vi "rsidr_core_global.vi"() -> ()   [LabVIEW 2020, in "Rohde&Schwarz RTx Oscilloscopes.lvlib"] (continued)
"Access"=2, "Range Table"="", "Read Callback"="", "Write Callback"="", "Supported Models"="", "Instrument Options"="", "Flags"=0, "Help"="If persistence is enabled (DISPlay:PERSistence[:STATe]), each new data point in the diagram area remains on the screen infinitely until this command is set to OFF.\n\nAvailable Repeated Capabilities:\nNone\n\nRemote-control command(s):\nDISPlay:PERSistence:INFinite"}, {"Level"=3, "Class Only"=FALSE, "Identifier"="RSRTX_ATTR_PERSISTENCE_TIME", "Descriptive Name"="Persistence Time", "Data Type"=1, "Command"="DISP:PERS:TIME", "Access"=2, "Range Table"="", "Read Callback"="", "Write Callback"="", "Supported Models"="", "Instrument Options"="", "Flags"=0, "Help"="If persistence is enabled (DISPlay:PERSistence[:STATe]), each new data point in the diagram area remains on the screen for the duration defined here.\n\nAvailable Repeated Capabilities:\nNone\n\nRemote-control command(s):\nDISPlay:PERSistence:TIME"}, {"Level"=3, "Class Only"=FALSE, "Identifier"="RSRTX_ATTR_PERSISTENCE_CLEAR", "Descriptive Name"="Persistence Clear", "Data Type"=4, "Command"="DISP:PERS:CLE", "Access"=1, "Range Table"="", "Read Callback"="", "Write Callback"="", "Supported Models"="", "Instrument Options"="", "Flags"=0, "Help"="Removes the displayed persistent waveform from the screen.\n\nAvailable Repeated Capabilities:\nNone\n\nRemote-control command(s):\nDISPlay:PERSistence:CLEar"}, {"Level"=2, "Class Only"=TRUE, "Identifier"="", "Descriptive Name"="XY Diagram", "Data Type"=0, "Command"="", "Access"=0, "Range Table"="", "Read Callback"="", "Write Callback"="", "Supported Models"="", "Instrument Options"="", "Flags"=0, "Help"="Contains attributes for XY Diagram settings."}, {"Level"=3, "Class Only"=FALSE, "Identifier"="RSRTX_ATTR_XY_X_SOURCE", "Descriptive Name"="XY X Source", "Data Type"=0, "Command"="DISP:XY:XSO", "Access"=2, "Range Table"="rsrtx_rngSource", "Read Callback"="", "Write Callback"="", "Supported Models"="", "Instrument Options"="", "Flags"=0, "Help"="Defines the source to be displayed in x direction in an XY-diagram, replacing the usual time base.\n\nAvailable Repeated Capabilities:\nNone\n\nRemote-control command(s):\nDISPlay:XY:XSOurce"}, {"Level"=3, "Class Only"=FALSE, "Identifier"="RSRTX_ATTR_XY_Y_SOURCE", "Descriptive Name"="XY Y Source", "Data Type"=0, "Command"="DISP:XY:Y1S", "Access"=2, "Range Table"="rsrtx_rngSource", "Read Callback"="", "Write Callback"="", "Supported Models"="", "Instrument Options"="", "Flags"=0, "Help"="Defines the (first) source to be displayed in y direction in an XY-diagram.\n\nAvailable Repeated Capabilities:\nNone\n\nRemote-control command(s):\nDISPlay:XY:Y1Source"}, {"Level"=3, "Class Only"=FALSE, "Identifier"="RSRTX_ATTR_XY_Y2_SOURCE", "Descriptive Name"="XY Y2 Source", "Data Type"=0, "Command"="DISP:XY:Y2S", "Access"=2, "Range Table"="rsrtx_rngXY2Source", "Read Callback"="", "Write Callback"="", "Supported Models"="", "Instrument Options"="", "Flags"=0, "Help"="Defines an optional second source to be displayed in y direction in an XY-diagram. Only relevant for 4-channel  instruments.\n\nAvailable Repeated Capabilities:\nNone\n\nRemote-control command(s):\nDISPlay:XY:Y2Source"}, {"Level"=3, "Class Only"=FALSE, "Identifier"="RSRTX_ATTR_XY_Z_SOURCE", "Descriptive Name"="XY Z Source", "Data Type"=0, "Command"="DISP:XY:ZSO", "Access"=2, "Range Table"="rsrtx_rngSource", "Read Callback"="", "Write Callback"="", "Supported Models"="", "Instrument Options"="", "Flags"=0, "Help"="Defines the source to be used to determine the intensity of the xy-waveform.\n\nAvailable Repeated Capabilities:\nNone\n\nRemote-control command(s):\nDISPlay:XY:ZSOurce"}, {"Level"=3, "Class Only"=FALSE, "Identifier"="RSRTX_ATTR_XY_Z_TRESHOLD", "Descriptive Name"="XY Z Treshold", "Data Type"=1, "Command"="DISP:XY:ZTHR", "Access"=2, "Range Table"="rsrtx_rngIntensityTreshold", "Read Callback"="", "Write Callback"="", "Supported Models"="", "Instrument Options"="", "Flags"=0, "Help"="Defines the threshold for intensity with a two-state modulation, if DISPlay: XY: ZMODe is set to DIGital.\n\nAvailable Repeated Capabilities:\nNone\n\nRemote-control command(s):\nDISPlay:XY:ZTHReshold"}, {"Level"=3, "Class Only"=FALSE, "Identifier"="RSRTX_ATTR_XY_INTENSITY_CONTROL", "Descriptive Name"="XY Intensity Control", "Data Type"=0, "Command"="DISP:XY:ZMOD", "Access"=2, "Range Table"="rsrtx_rngIntensityMode", "Read Callback"="", "Write Callback"="", "Supported Models"="", "Instrument Options"="", "Flags"=0, "Help"="Activates or deactivates the intensity control of the waveform via an additional signal source and sets the intensity mode.\n\nAvailable Repeated Capabilities:\nNone\n\nRemote-control command(s):\nDISPlay:XY:ZMODe"}, {"Level"=2, "Class Only"=TRUE, "Identifier"="", "Descriptive Name"="Zoom", "Data Type"=0, "Command"="", "Access"=0, "Range Table"="", "Read Callback"="", "Write Callback"="", "Supported Models"="", "Instrument Options"="", "Flags"=0, "Help"="Zoom definition."}, {"Level"=3, "Class Only"=FALSE, "Identifier"="RSRTX_ATTR_ZOOM_WINDOW_ENABLED", "Descriptive Name"="Zoom Window Enabled", "Data Type"=3, "Command"="TIM:ZOOM:STAT", "Access"=2, "Range Table"="", "Read Callback"="", "Write Callback"="", "Supported Models"="", "Instrument Options"="", "Flags"=0, "Help"="Switches the zoom window on or off.\n\nAvailable Repeated Capabilities:\nNone\n\nRemote-control command(s):\nTIMebase:ZOOM:STATe"}, {"Level"=3, "Class Only"=FALSE, "Identifier"="RSRTX_ATTR_ZOOM_DIAGRAM_TIMEBASE", "Descriptive Name"="Zoom Diagram Timebase", "Data Type"=1, "Command"="TIM:ZOOM:SCAL", "Access"=2, "Range Table"="", "Read Callback"="", "Write Callback"="", "Supported Models"="", "Instrument Options"="", "Flags"=0, "Help"="Defines the time base in the zoom diagram in seconds per division.\n\nAvailable Repeated Capabilities:\nNone\n\nRemote-control command(s):\nTIMebase:ZOOM:SCALe"}, {"Level"=3, "Class Only"=FALSE, "Identifier"="RSRTX_ATTR_ZOOM_OFFSET_OF_TRIGGER_POINT", "Descriptive Name"="Zoom Offset Of Trigger Point", "Data Type"=1, "Command"="TIM:ZOOM:TIME", "Access"=2, "Range Table"="", "Read Callback"="", "Write Callback"="", "Supported Models"="", "Instrument Options"="", "Flags"=0, "Help"="Defines the offset of the trigger point to the reference point of the zoom diagram.\n\nAvailable Repeated Capabilities:\nNone\n\nRemote-control command(s):\nTIMebase:ZOOM:TIME"}, {"Level"=3, "Class Only"=FALSE, "Identifier"="RSRTX_ATTR_ZOOM_REFERENCE_POINT", "Descriptive Name"="Zoom Reference Point", "Data Type"=1, "Command"="TIM:ZOOM:POS", "Access"=2, "Range Table"="rsrtx_rngPct", "Read Callback"="", "Write Callback"="", "Supported Models"="", "Instrument Options"="", "Flags"=0, "Help"="Defines the position of the zoom reference point (the reference point of the zoom window) in relation to the reference point of original time base.\n\nAvailable Repeated Capabilities:\nNone\n\nRemote-control command(s):\nTIMebase:ZOOM:POSition"}, {"Level"=3, "Class Only"=FALSE, "Identifier"="RSRTX_ATTR_ZOOM_WINDOW_POSITION", "Descriptive Name"="Zoom Window Position", "Data Type"=0, "Command"="DISP:CBAR:ZOOM", "Access"=2, "Range Table"="", "Read Callback"="", "Write Callback"="", "Supported Models"="", "Instrument Options"="", "Flags"=0, "Help"="Defines the position of the divide bar between normal waveform and zoom window. Sets the vertical position in pixels, measured from the top edge. The vertical display size is 800 px.\n\nAvailable Repeated Capabilities:\nNone\n\nRemote-control command(s):\nDISPlay:CBAR:ZOOM[:POSition]"}, {"Level"=3, "Class Only"=FALSE, "Identifier"="RSRTX_ATTR_ZOOM_SAMPLE_RATE", "Descriptive Name"="Zoom Sample Rate", "Data Type"=1, "Command"="ACQ:SRAT:ZOOM?", "Access"=0, "Range Table"="", "Read Callback"="", "Write Callback"="", "Supported Models"="", "Instrument Options"="", "Flags"=0, "Help"="Returns the sample rate of the zoom window.\n\nAvailable Repeated Capabilities:\nNone\n\nRemote-control command(s):\nACQuire:SRATe:ZOOM?"}, {"Level"=2, "Class Only"=TRUE, "Identifier"="", "Descriptive Name"="Markers", "Data Type"=0, "Command"="", "Access"=0, "Range Table"="", "Read Callback"="", "Write Callback"="", "Supported Models"="", "Instrument Options"="", "Flags"=0, "Help"="Markers configuration."}, {"Level"=3, "Class Only"=FALSE, "Identifier"="RSRTX_ATTR_MARKER_SET", "Descriptive Name"="Marker Set", "Data Type"=4, "Command"="TST:SET", "Access"=1, "Range Table"="", "Read Callback"="", "Write Callback"="", "Supported Models"="", "Instrument Options"="", "Flags"=0, "Help"="Sets a new marker (timestamp) at the reference point of the display, unless an existing marker is already set there. The reference point is set with RSRTX_ATTR_HORZ_REFERENCE.\n\nAvailable Repeated Capabilities:\nNone\n\nRemote-control command(s):\nTSTamp:SET"}, {"Level"=3, "Class Only"=FALSE, "Identifier"="RSRTX_ATTR_MARKER_CLEAR", "Descriptive Name"="Marker Clear", "Data Type"=4, "Command"="TST:CLE", "Access"=1, "Range Table"="", "Read Callback"="", "Write Callback"="", "Supported Models"="", "Instrument Options"="", "Flags"=0, "Help"="Deletes the marker (timestamp) at the reference point. The reference point is set with TIMebase: REFerence.\n\nAvailable Repeated Capabilities:\nNone\n\nRemote-control command(s):\nTSTamp:CLEar"}, {"Level"=3, "Class Only"=FALSE, "Identifier"="RSRTX_ATTR_MARKER_CLEAR_ALL", "Descriptive Name"="Marker Clear All", "Data Type"=4, "Command"="TST:ACL", "Access"=1, "Range Table"="", "Read Callback"="", "Write Callback"="", "Supported Models"="", "Instrument Options"="", "Flags"=0, "Help"="Deletes all markers (timestamps).\n\nAvailable Repeated Capabilities:\nNone\n\nRemote-control command(s):\nTSTamp:ACLear"}, {"Level"=3, "Class Only"=FALSE, "Identifier"="RSRTX_ATTR_MARKER_NEXT", "Descriptive Name"="Marker Next", "Data Type"=4, "Command"="TST:NEXT", "Access"=1, "Range Table"="", "Read Callback"="", "Write Callback"="", "Supported Models"="", "Instrument Options"="", "Flags"=0, "Help"="Moves the next marker (timestamp, to the right) to the reference point of the display or zoom area.\n\nAvailable Repeated Capabilities:\nNone\n\nRemote-control command(s):\nTSTamp:NEXT"}, {"Level"=3, "Class Only"=FALSE, "Identifier"="RSRTX_ATTR_MARKER_PREVIOUS", "Descriptive Name"="Marker Previous", "Data Type"=4, "Command"="TST:PREV", "Access"=1, "Range Table"="", "Read Callback"="", "Write Callback"="", "Supported Models"="", "Instrument Options"="", "Flags"=0, "Help"="Moves the previous marker (timestamp, to the left) to the reference point of the display or zoom area.\n\nAvailable Repeated Capabilities:\nNone\n\nRemote-control command(s):\nTSTamp:PREVious"}, {"Level"=2, "Class Only"=TRUE, "Identifier"="", "Descriptive Name"="Virtual Screen", "Data Type"=0, "Command"="", "Access"=0, "Range Table"="", "Read Callback"="", "Write Callback"="", "Supported Models"="", "Instrument Options"="", "Flags"=0, "Help"="Contains attributes for Virtual Screen."}, {"Level"=3, "Class Only"=FALSE, "Identifier"="RSRTX_ATTR_VIRTUAL_SCREEN_ENABLED", "Descriptive Name"="Virtual Screen Enabled", "Data Type"=3, "Command"="DISP:VSCR:ENAB", "Access"=2, "Range Table"="", "Read Callback"="", "Write Callback"="", "Supported Models"="", "Instrument Options"="", "Flags"=0, "Help"="Enables or disables the virtual screen. If enabled, the virtual screen has 20 divisions, 8 of them are displayed.\n\nAvailable Repeated Capabilities:\nNone\n\nRemote-control command(s):\nDISPlay:VSCReen:ENABle"}, {"Level"=3, "Class Only"=FALSE, "Identifier"="RSRTX_ATTR_VIRTUAL_SCREEN_POSITION", "Descriptive Name"="Virtual Screen Position", "Data Type"=1, "Command"="DISP:VSCR:POS", "Access"=2, "Range Table"="", "Read Callback"="", "Write Callback"="", "Supported Models"="", "Instrument Options"="", "Flags"=0, "Help"="Selects the divisions to be displayed on the virtual screen. The virtual screen has 20 divisions, 8 of them are displayed.\n\nAvailable Repeated Capabilities:\nNone\n\nRemote-control command(s):\nDISPlay:VSCReen:POSition"}, {"Level"=2, "Class Only"=TRUE, "Identifier"="", "Descriptive Name"="History", "Data Type"=0, "Command"="", "Access"=0, "Range Table"="", "Read Callback"="", "Write Callback"="", "Supported Models"="", "Instrument Options"="", "Flags"=0, "Help"="Configures history."}, {"Level"=3, "Class Only"=TRUE, "Identifier"="", "Descriptive Name"="Channel", "Data Type"=0, "Command"="", "Access"=0, "Range Table"="", "Read Callback"="", "Write Callback"="", "Supported Models"="", "Instrument Options"="", "Flags"=0, "Help"="Configures history for channel"}, {"Level"=4, "Class Only"=FALSE, "Identifier"="RSRTX_ATTR_HISTORY_CHANNEL_CURRENT_ACQUISITION", "Descriptive Name"="History Channel Current Acquisition", "Data Type"=0, "Command"="CHAN{Channel}:HIST:CURR", "Access"=2, "Range Table"="", "Read Callback"="", "Write Callback"="", "Supported Models"="", "Instrument Options"="K15", "Flags"=0, "Help"="Accesses a particular acquisition segment in the memory to display it. The query returns the index of the segment that is shown.\nThere are two ways to enter the index.\nNegative index count: the newest segment has the index 0, older segments have a negative index: -(n-1), .... -1 , 0\nPositive index count: the oldest segment has the index 1, and the newest segment has the index n: 1, 2,..., n\nwhere n is the number of acquired segments.\n\nAvailable Repeated Capabilities:\nChannel: CH0, CH1, CH2, CH3, CH4, CHExt\r\n\nRemote-control command(s):\nCHANnel<m>:HISTory:CURRent"}, {"Level"=4, "Class Only"=FALSE, "Identifier"="RSRTX_ATTR_HISTORY_CHANNEL_PLAYER", "Descriptive Name"="History Channel Player", "Data Type"=0, "Command"="CHAN{Channel}:HIST:PLAY:STAT", "Access"=2, "Range Table"="rsrtx_rngHistoryPlayer", "Read Callback"="", "Write Callback"="", "Supported Models"="", "Instrument Options"="K15", "Flags"=0, "Help"="Starts and stops the replay of the history segments.\n\nAvailable Repeated Capabilities:\nChannel: CH0, CH1, CH2, CH3, CH4, CHExt\r\n\nRemote-control command(s):\nCHANnel<m>:HISTory:PLAYer:STATe"}, {"Level"=4, "Class Only"=FALSE, "Identifier"="RSRTX_ATTR_HISTORY_CHANNEL_START_ACQUISITION", "Descriptive Name"="History Channel Start Acquisition", "Data Type"=0, "Command"="CHAN{Channel}:HIST:STAR", "Access"=2, "Range Table"="", "Read Callback"="", "Write Callback"="", "Supported Models"="", "Instrument Options"="K15", "Flags"=0, "Help"="Sets the index of the oldest segment to be displayed.\nThere are two ways to enter the index.\nNegative index count: the newest segment has the index 0, older segments have a negative index: -(n-1), .... -1 , 0\nPositive index count: the oldest segment has the index 1, and the newest segment has the index n: 1, 2,..., n\nwhere n is the number of acquired segments.\n\nAvailable Repeated Capabilities:\nChannel: CH0, CH1, CH2, CH3, CH4, CHExt\r\n\nRemote-control command(s):\nCHANnel<m>:HISTory:STARt"}, {"Level"=4, "Class Only"=FALSE, "Identifier"="RSRTX_ATTR_HISTORY_CHANNEL_STOP_ACQUISITION", "Descriptive Name"="History Channel Stop Acquisition", "Data Type"=0, "Command"="CHAN{Channel}:HIST:STOP", "Access"=2, "Range Table"="", "Read Callback"="", "Write Callback"="", "Supported Models"="", "Instrument Options"="K15", "Flags"=0, "Help"="Sets the index of the latest segment to be displayed.\nThere are two ways to enter the index.\nNegative index count: the newest segment has the index 0, older segments have a negative index: -(n-1), .... -1 , 0\nPositive index count: the oldest segment has the index 1, and the newest segment has the index n: 1, 2,..., n\nwhere n is the number of acquired segments.\n\nAvailable Repeated Capabilities:\nChannel: CH0, CH1, CH2, CH3, CH4, CHExt\r\n\nRemote-control command(s):\nCHANnel<m>:HISTory:STOP"}, {"Level"=4, "Class Only"=FALSE, "Identifier"="RSRTX_ATTR_HISTORY_CHANNEL_PLAY_ALL", "Descriptive Name"="History Channel Play All", "Data Type"=3, "Command"="CHAN{Channel}:HIST:PALL", "Access"=2, "Range Table"="", "Read Callback"="", "Write Callback"="", "Supported Models"="", "Instrument Options"="K15", "Flags"=0, "Help"="Enables the replay of all acquired segments.\n\nAvailable Repeated Capabilities:\nChannel: CH0, CH1, CH2, CH3, CH4, CHExt\r\n\nRemote-control command(s):\nCHANnel<m>:HISTory:PALL"}, {"Level"=4, "Class Only"=FALSE, "Identifier"="RSRTX_ATTR_HISTORY_CHANNEL_SPEED", "Descriptive Name"="History Channel Speed", "Data Type"=0, "Command"="CHAN{Channel}:HIST:PLAY:SPE", "Access"=2, "Range Table"="rsrtx_rngHistorySpeed", "Read Callback"="", "Write Callback"="", "Supported Models"="", "Instrument Options"="K15", "Flags"=0, "Help"="Sets the speed of the history replay.\n\nAvailable Repeated Capabilities:\nChannel: CH0, CH1, CH2, CH3, CH4, CHExt\r\n\nRemote-control command(s):\nCHANnel<m>:HISTory:PLAYer:SPEed"}, {"Level"=4, "Class Only"=FALSE, "Identifier"="RSRTX_ATTR_HISTORY_CHANNEL_REPEAT", "Descriptive Name"="History Channel Repeat", "Data Type"=3, "Command"="CHAN{Channel}:HIST:REPL", "Access"=2, "Range Table"="", "Read Callback"="", "Write Callback"="", "Supported Models"="", "Instrument Options"="K15", "Flags"=0, "Help"="If set to true, the replay of the selected history segments repeats automatically.\n\nAvailable Repeated Capabilities:\nChannel: CH0, CH1, CH2, CH3, CH4, CHExt\r\n\nRemote-control command(s):\nCHANnel<m>:HISTory:REPLay"}, {"Level"=4, "Class Only"=FALSE, "Identifier"="RSRTX_ATTR_HISTORY_CHANNEL_ACQUISITON_RELATIVE_TIME", "Descriptive Name"="History Channel Acquisiton Relative Time", "Data Type"=1, "Command"="CHAN{Channel}:HIST:TSR?", "Access"=0, "Range Table"="", "Read Callback"="", "Write Callback"="", "Supported Models"="", "Instrument Options"="K15", "Flags"=0, "Help"="Returns the time difference of the selected segment to the newest segment.\n\nAvailable Repeated Capabilities:\nChannel: CH0, CH1, CH2, CH3, CH4, CHExt\r\n\nRemote-control command(s):\nCHANnel<m>:HISTory:TSRelative?"}, {"Level"=4, "Class Only"=FALSE, "Identifier"="RSRTX_ATTR_HISTORY_CHANNEL_ALL_DATES", "Descriptive Name"="History Channel All Dates", "Data Type"=2, "Command"="CHAN{Channel}:HIST:TSD:ALL?", "Access"=0, "Range Table"="", "Read Callback"="", "Write Callback"="", "Supported Models"="", "Instrument Options"="", "Flags"=0, "Help"="Returns the dates of all history segments.\n\nAvailable Repeated Capabilities:\nChannel: CH0, CH1, CH2, CH3, CH4, CHExt\r\n\nRemote-control command(s):\nCHANnel<m>:HISTory:TSDate:ALL?"}, {"Level"=4, "Class Only"=FALSE, "Identifier"="RSRTX_ATTR_HISTORY_CHANNEL_ALL_TIME_DIFFERENCES", "Descriptive Name"="History Channel All Time Differences", "Data Type"=2, "Command"="CHAN{Channel}:HIST:TSR:ALL?", "Access"=0, "Range Table"="", "Read Callback"="", "Write Callback"="", "Supported Models"="", "Instrument Options"="", "Flags"=0, "Help"="Returns the time differences to the newest acquisition of all history segments.\n\nAvailable Repeated Capabilities:\nChannel: CH0, CH1, CH2, CH3, CH4, CHExt\r\n\nRemote-control command(s):\nCHANnel<m>:HISTory:TSRelative:ALL?"}, {"Level"=4, "Class Only"=FALSE, "Identifier"="RSRTX_ATTR_HISTORY_CHANNEL_ALL_DAYTIMES", "Descriptive Name"="History Channel All Daytimes", "Data Type"=2, "Command"="CHAN{Channel}:HIST:TSAB:ALL?", "Access"=0, "Range Table"="", "Read Callback"="", "Write Callback"="", "Supported Models"="", "Instrument Options"="", "Flags"=0, "Help"="Returns the absolute daytimes of all history segments.\n\nAvailable Repeated Capabilities:\nChannel: CH0, CH1, CH2, CH3, CH4, CHExt\r\n\nRemote-control command(s):\nCHANnel<m>:HISTory:TSABsolute:ALL?"}, {"Level"=4, "Class Only"=FALSE, "Identifier"="RSRTX_ATTR_HISTORY_CHANNEL_PLAYER_CONTROL_ENABLE", "Descriptive Name"="History Channel Player Control Enable", "Data Type"=3, "Command"="CHAN{Channel}:HIST:CONT", "Access"=2, "Range Table"="", "Read Callback"="", "Write Callback"="", "Supported Models"="", "Instrument Options"="K15", "Flags"=0, "Help"="Displays or hides the history player on the screen.\n\nAvailable Repeated Capabilities:\nChannel: CH0, CH1, CH2, CH3, CH4, CHExt\r\n\nRemote-control command(s):\nCHANnel<m>:HISTory:CONTrol:[ENABle]"}, {"Level"=4, "Class Only"=FALSE, "Identifier"="RSRTX_ATTR_HISTORY_CHANNEL_TABLE_MODE", "Descriptive Name"="History Channel Table Mode", "Data Type"=0, "Command"="CHAN{Channel}:HIST:TMOD?", "Access"=0, "Range Table"="RsRtx_rngAbsoluteRelative", "Read Callback"="", "Write Callback"="", "Supported Models"="", "Instrument Options"="", "Flags"=0, "Help"="Returns the the type of the timestamp that is shown the segment table.\n\nAvailable Repeated Capabilities:\nChannel: CH0, CH1, CH2, CH3, CH4, CHExt\r\n\nRemote-control command(s):\nCHANnel<m>:HISTory:TMODe?"}, {"Level"=4, "Class Only"=FALSE, "Identifier"="RSRTX_ATTR_HISTORY_CHANNEL_TIME_TABLE_ENABLE", "Descriptive Name"="History Channel Time Table Enable", "Data Type"=3, "Command"="CHAN{Channel}:HIST:TTAB", "Access"=2, "Range Table"="", "Read Callback"="", "Write Callback"="", "Supported Models"="", "Instrument Options"="K15", "Flags"=0, "Help"="Displays or hides the segment table on the screen.\n\nAvailable Repeated Capabilities:\nChannel: CH0, CH1, CH2, CH3, CH4, CHExt\r\n\nRemote-control command(s):\nCHANnel<m>:HISTory:TTABle[:ENABle]"}, {"Level"=4, "Class Only"=FALSE, "Identifier"="RSRTX_ATTR_HISTORY_CHANNEL_EXPORT_NAME", "Descriptive Name"="History Channel Export Name", "Data Type"=2, "Command"="CHAN{Channel}:HIST:EXP:NAME", "Access"=2, "Range Table"="", "Read Callback"="", "Write Callback"="", "Supported Models"="", "Instrument Options"="", "Flags"=0, "Help"="Configures export file name.\n\nAvailable Repeated Capabilities:\nChannel: CH0, CH1, CH2, CH3, CH4, CHExt\r\n\nRemote-control command(s):\nCHANnel<m>:HISTory:EXPort:NAME"}, {"Level"=4, "Class Only"=FALSE, "Identifier"="RSRTX_ATTR_HISTORY_CHANNEL_EXPORT_SAVE", "Descriptive Name"="History Channel Export Save", "Data Type"=4, "Command"="CHAN{Channel}:HIST:EXP:SAVE", "Access"=1, "Range Table"="", "Read Callback"="", "Write Callback"="", "Supported Models"="", "Instrument Options"="", "Flags"=0, "Help"="Exports channel history.\n\nAvailable Repeated Capabilities:\nChannel: CH0, CH1, CH2, CH3, CH4, CHExt\r\n\nRemote-control command(s):\nCHANnel<m>:HISTory:EXPort:SAVE"}, {"Level"=3, "Class Only"=TRUE, "Identifier"="", "Descriptive Name"="Digital", "Data Type"=0, "Command"="", "Access"=0, "Range Table"="", "Read Callback"="", "Write Callback"="", "Supported Models"="", "Instrument Options"="", "Flags"=0, "Help"="Configures history for digital channel"}, {"Level"=4, "Class Only"=FALSE, "Identifier"="RSRTX_ATTR_HISTORY_DIGITAL_CURRENT_ACQUISITION", "Descriptive Name"="History Digital Current Acquisition", "Data Type"=0, "Command"="DIG{Digital}:HIST:CURR", "Access"=2, "Range Table"="", "Read Callback"="", "Write Callback"="", "Supported Models"="", "Instrument Options"="K15", "Flags"=0, "Help"="Accesses a particular acquisition segment in the memory to display it. The query returns the index of the segment that is shown.\nThere are two ways to enter the index.\nNegative index count: the newest segment has the index 0, older segments have a negative index: -(n-1), .... -1 , 0\nPositive index count: the oldest segment has the index 1, and the newest segment has the index n: 1, 2,..., n\nwhere n is the number of acquired segments.\n\nAvailable Repeated Capabilities:\nDigital: D0, D1, D2, D3, D4, D5, D6, D7, D8, D9, D10, D11, D12, D13, D14, D15\r\n\nRemote-control command(s):\nDIGital<m>:HISTory:CURRent"}, {"Level"=4, "Class Only"=FALSE, "Identifier"="RSRTX_ATTR_HISTORY_DIGITAL_PLAYER", "Descriptive Name"="History Digital Player", "Data Type"=0, "Command"="DIG{Digital}:HIST:PLAY:STAT", "Access"=2, "Range Table"="rsrtx_rngHistoryPlayer", "Read Callback"="", "Write Callback"="", "Supported Models"="", "Instrument Options"="K15", "Flags"=0, "Help"="Starts and stops the replay of the history segments.\n\nAvailable Repeated Capabilities:\nDigital: D0, D1, D2, D3, D4, D5, D6, D7, D8, D9, D10, D11, D12, D13, D14, D15\r\n\nRemote-control command(s):\nDIGital<m>:HISTory:PLAYer:STATe"}, {"Level"=4, "Class Only"=FALSE, "Identifier"="RSRTX_ATTR_HISTORY_DIGITAL_START_ACQUISITION", "Descriptive Name"="History Digital Start Acquisition", "Data Type"=0, "Command"="DIG{Digital}:HIST:STAR", "Access"=2, "Range Table"="", "Read Callback"="", "Write Callback"="", "Supported Models"="", "Instrument Options"="K15", "Flags"=0, "Help"="Sets the index of the oldest segment to be displayed.\nThere are two ways to enter the index.\nNegative index count: the newest segment has the index 0, older segments have a negative index: -(n-1), .... -1 , 0\nPositive index count: the oldest segment has the index 1, and the newest segment has the index n: 1, 2,..., n\nwhere n is the number of acquired segments.\n\nAvailable Repeated Capabilities:\nDigital: D0, D1, D2, D3, D4, D5, D6, D7, D8, D9, D10, D11, D12, D13, D14, D15\r\n\nRemote-control command(s):\nDIGital<m>:HISTory:STARt"}, {"Level"=4, "Class Only"=FALSE, "Identifier"="RSRTX_ATTR_HISTORY_DIGITAL_STOP_ACQUISITION", "Descriptive Name"="History Digital Stop Acquisition", "Data Type"=0, "Command"="DIG{Digital}:HIST:STOP", "Access"=2, "Range Table"="", "Read Callback"="", "Write Callback"="", "Supported Models"="", "Instrument Options"="K15", "Flags"=0, "Help"="Sets the index of the latest segment to be displayed.\nThere are two ways to enter the index.\nNegative index count: the newest segment has the index 0, older segments have a negative index: -(n-1), .... -1 , 0\nPositive index count: the oldest segment has the index 1, and the newest segment has the index n: 1, 2,..., n\nwhere n is the number of acquired segments.\n\nAvailable Repeated Capabilities:\nDigital: D0, D1, D2, D3, D4, D5, D6, D7, D8, D9, D10, D11, D12, D13, D14, D15\r\n\nRemote-control command(s):\nDIGital<m>:HISTory:STOP"}, {"Level"=4, "Class Only"=FALSE, "Identifier"="RSRTX_ATTR_HISTORY_DIGITAL_PLAY_ALL", "Descriptive Name"="History Digital Play All", "Data Type"=3, "Command"="DIG{Digital}:HIST:PALL", "Access"=2, "Range Table"="", "Read Callback"="", "Write Callback"="", "Supported Models"="", "Instrument Options"="K15", "Flags"=0, "Help"="Enables the replay of all acquired segments.\n\nAvailable Repeated Capabilities:\nDigital: D0, D1, D2, D3, D4, D5, D6, D7, D8, D9, D10, D11, D12, D13, D14, D15\r\n\nRemote-control command(s):\nDIGital<m>:HISTory:PALL"}, {"Level"=4, "Class Only"=FALSE, "Identifier"="RSRTX_ATTR_HISTORY_DIGITAL_SPEED", "Descriptive Name"="History Digital Speed", "Data Type"=0, "Command"="DIG{Digital}:HIST:PLAY:SPE", "Access"=2, "Range Table"="rsrtx_rngHistorySpeed", "Read Callback"="", "Write Callback"="", "Supported Models"="", "Instrument Options"="K15", "Flags"=0, "Help"="Sets the speed of the history replay.\n\nAvailable Repeated Capabilities:\nDigital: D0, D1, D2, D3, D4, D5, D6, D7, D8, D9, D10, D11, D12, D13, D14, D15\r\n\nRemote-control command(s):\nDIGital<m>:HISTory:PLAYer:SPEed"}, {"Level"=4, "Class Only"=FALSE, "Identifier"="RSRTX_ATTR_HISTORY_DIGITAL_REPEAT", "Descriptive Name"="History Digital Repeat", "Data Type"=3, "Command"="DIG{Digital}:HIST:REPL", "Access"=2, "Range Table"="", "Read Callback"="", "Write Callback"="", "Supported Models"="", "Instrument Options"="K15", "Flags"=0, "Help"="If set to true, the replay of the selected history segments repeats automatically.\n\nAvailable Repeated Capabilities:\nDigital: D0, D1, D2, D3, D4, D5, D6, D7, D8, D9, D10, D11, D12, D13, D14, D15\r\n\nRemote-control command(s):\nDIGital<m>:HISTory:REPLay"}, {"Level"=4, "Class Only"=FALSE, "Identifier"="RSRTX_ATTR_HISTORY_DIGITAL_ACQUISITON_RELATIVE_TIME", "Descriptive Name"="History Digital Acquisiton Relative Time", "Data Type"=1, "Command"="DIG{Digital}:HIST:TSR?", "Access"=0, "Range Table"="", "Read Callback"="", "Write Callback"="", "Supported Models"="", "Instrument Options"="K15", "Flags"=0, "Help"="Returns the time difference of the selected segment to the newest segment.\n\nAvailable Repeated Capabilities:\nDigital: D0, D1, D2, D3, D4, D5, D6, D7, D8, D9, D10, D11, D12, D13, D14, D15\r\n\nRemote-control command(s):\nDIGital<m>:HISTory:TSRelative?"}, {"Level"=4, "Class Only"=FALSE, "Identifier"="RSRTX_ATTR_HISTORY_DIGITAL_ALL_DATES", "Descriptive Name"="History Digital All Dates", "Data Type"=2, "Command"="DIG{Digital}:HIST:TSD:ALL?", "Access"=0, "Range Table"="", "Read Callback"="", "Write Callback"="", "Supported Models"="", "Instrument Options"="", "Flags"=0, "Help"="Returns the dates of all history segments.\n\nAvailable Repeated Capabilities:\nDigital: D0, D1, D2, D3, D4, D5, D6, D7, D8, D9, D10, D11, D12, D13, D14, D15\r\n\nRemote-control command(s):\nDIGital<m>:HISTory:TSDate:ALL?"}, {"Level"=4, "Class Only"=FALSE, "Identifier"="RSRTX_ATTR_HISTORY_DIGITAL_ALL_TIME_DIFFERENCES", "Descriptive Name"="History Digital All Time Differences", "Data Type"=2, "Command"="DIG{Digital}:HIST:TSR:ALL?", "Access"=0, "Range Table"="", "Read Callback"="", "Write Callback"="", "Supported Models"="", "Instrument Options"="", "Flags"=0, "Help"="Returns the time differences to the newest acquisition of all history segments.\n\nAvailable Repeated Capabilities:\nDigital: D0, D1, D2, D3, D4, D5, D6, D7, D8, D9, D10, D11, D12, D13, D14, D15\r\n\nRemote-control command(s):\nDIGital<m>:HISTory:TSRelative:ALL?"}, {"Level"=4, "Class Only"=FALSE, "Identifier"="RSRTX_ATTR_HISTORY_DIGITAL_ALL_DAYTIMES", "Descriptive Name"="History Digital All Daytimes", "Data Type"=2, "Command"="DIG{Digital}:HIST:TSAB:ALL?", "Access"=0, "Range Table"="", "Read Callback"="", "Write Callback"="", "Supported Models"="", "Instrument Options"="", "Flags"=0, "Help"="Returns the absolute daytimes of all history segments.\n\nAvailable Repeated Capabilities:\nDigital: D0, D1, D2, D3, D4, D5, D6, D7, D8, D9, D10, D11, D12, D13, D14, D15\r\n\nRemote-control command(s):\nDIGital<m>:HISTory:TSABsolute:ALL?"}, {"Level"=4, "Class Only"=FALSE, "Identifier"="RSRTX_ATTR_HISTORY_DIGITAL_PLAYER_CONTROL_ENABLE", "Descriptive Name"="History Digital Player Control Enable", "Data Type"=3, "Command"="DIG{Digital}:HIST:CONT", "Access"=2, "Range Table"="", "Read Callback"="", "Write Callback"="", "Supported Models"="", "Instrument Options"="K15", "Flags"=0, "Help"="Displays or hides the history player on the screen.\n\nAvailable Repeated Capabilities:\nDigital: D0, D1, D2, D3, D4, D5, D6, D7, D8, D9, D10, D11, D12, D13, D14, D15\r\n\nRemote-control command(s):\nDIGital<m>:HISTory:CONTrol[:ENABle]"}, {"Level"=4, "Class Only"=FALSE, "Identifier"="RSRTX_ATTR_HISTORY_DIGITAL_TIME_TABLE_ENABLE", "Descriptive Name"="History Digital Time Table Enable", "Data Type"=3, "Command"="DIG{Digital}:HIST:TTAB", "Access"=2, "Range Table"="", "Read Callback"="", "Write Callback"="", "Supported Models"="", "Instrument Options"="K15", "Flags"=0, "Help"="Displays or hides the segment table on the screen.\n\nAvailable Repeated Capabilities:\nDigital: D0, D1, D2, D3, D4, D5, D6, D7, D8, D9, D10, D11, D12, D13, D14, D15\r\n\nRemote-control command(s):\nDIGital<m>:HISTory:TTABle[:ENABle]"}, {"Level"=4, "Class Only"=FALSE, "Identifier"="RSRTX_ATTR_DIGITAL_HISTORY_EXPORT_NAME", "Descriptive Name"="Digital History Export Name", "Data Type"=2, "Command"="DIG{Digital}:HIST:EXP:NAME", "Access"=2, "Range Table"="", "Read Callback"="", "Write Callback"="", "Supported Models"="", "Instrument Options"="", "Flags"=0, "Help"="Configures export file name.\n\nAvailable Repeated Capabilities:\nDigital: D0, D1, D2, D3, D4, D5, D6, D7, D8, D9, D10, D11, D12, D13, D14, D15\r\n\nRemote-control command(s):\nDIGital<m>:HISTory:EXPort:NAME"}, {"Level"=4, "Class Only"=FALSE, "Identifier"="RSRTX_ATTR_DIGITAL_HISTORY_EXPORT_SAVE", "Descriptive Name"="Digital History Export Save", "Data Type"=4, "Command"="DIG{Digital}:HIST:EXP:SAVE", "Access"=1, "Range Table"="", "Read Callback"="", "Write Callback"="", "Supported Models"="", "Instrument Options"="", "Flags"=0, "Help"="Exports channel history.\n\nAvailable Repeated Capabilities:\nDigital: D0, D1, D2, D3, D4, D5, D6, D7, D8, D9, D10, D11, D12, D13, D14, D15\r\n\nRemote-control command(s):\nDIGital<m>:HISTory:EXPort:SAVE"}, {"Level"=3, "Class Only"=TRUE, "Identifier"="", "Descriptive Name"="Math", "Data Type"=0, "Command"="", "Access"=0, "Range Table"="", "Read Callback"="", "Write Callback"="", "Supported Models"="", "Instrument Options"="", "Flags"=0, "Help"="Configures history for math channel"}, {"Level"=4, "Class Only"=FALSE, "Identifier"="RSRTX_ATTR_HISTORY_MATH_CURRENT_ACQUISITION", "Descriptive Name"="History Math Current Acquisition", "Data Type"=0, "Command"="CALC:MATH{Math}:HIST:CURR", "Access"=2, "Range Table"="", "Read Callback"="", "Write Callback"="", "Supported Models"="RTM|RTA", "Instrument Options"="K15", "Flags"=0, "Help"="Accesses a particular acquisition segment in the memory to display it. The query returns the index of the segment that is shown.\nThere are two ways to enter the index.\nNegative index count: the newest segment has the index 0, older segments have a negative index: -(n-1), .... -1 , 0\nPositive index count: the oldest segment has the index 1, and the newest segment has the index n: 1, 2,..., n\nwhere n is the number of acquired segments.\n\nAvailable Repeated Capabilities:\nMath: MA1, MA2, MA3, MA4, MA5\r\n\nRemote-control command(s):\nCALCulate:MATH<m>:HISTory:CURRent"}, {"Level"=4, "Class Only"=FALSE, "Identifier"="RSRTX_ATTR_HISTORY_MATH_PLAYER", "Descriptive Name"="History Math Player", "Data Type"=0, "Command"="CALC:MATH{Math}:HIST:PLAY:STAT", "Access"=2, "Range Table"="rsrtx_rngHistoryPlayer", "Read Callback"="", "Write Callback"="", "Supported Models"="RTM|RTA", "Instrument Options"="K15", "Flags"=0, "Help"="Starts and stops the replay of the history segments.\n\nAvailable Repeated Capabilities:\nMath: MA1, MA2, MA3, MA4, MA5\r\n\nRemote-control command(s):\nCALCulate:MATH<m>:HISTory:PLAYer:STATe"}, {"Level"=4, "Class Only"=FALSE, "Identifier"="RSRTX_ATTR_HISTORY_MATH_START_ACQUISITION", "Descriptive Name"="History Math Start Acquisition", "Data Type"=0, "Command"="CALC:MATH{Math}:HIST:STAR", "Access"=2, "Range Table"="", "Read Callback"="", "Write Callback"="", "Supported Models"="RTM|RTA", "Instrument Options"="K15", "Flags"=0, "Help"="Sets the index of the oldest segment to be displayed.\nThere are two ways to enter the index.\nNegative index count: the newest segment has the index 0, older segments have a negative index: -(n-1), .... -1 , 0\nPositive index count: the oldest segment has the index 1, and the newest segment has the index n: 1, 2,..., n\nwhere n is the number of acquired segments.\n\nAvailable Repeated Capabilities:\nMath: MA1, MA2, MA3, MA4, MA5\r\n\nRemote-control command(s):\nCALCulate:MATH<m>:HISTory:STARt"}, {"Level"=4, "Class Only"=FALSE, "Identifier"="RSRTX_ATTR_HISTORY_MATH_STOP_ACQUISITION", "Descriptive Name"="History Math Stop Acquisition", "Data Type"=0, "Command"="CALC:MATH{Math}:HIST:STOP", "Access"=2, "Range Table"="", "Read Callback"="", "Write Callback"="", "Supported Models"="RTM|RTA", "Instrument Options"="K15", "Flags"=0, "Help"="Sets the index of the latest segment to be displayed.\nThere are two ways to enter the index.\nNegative index count: the newest segment has the index 0, older segments have a negative index: -(n-1), .... -1 , 0\nPositive index count: the oldest segment has the index 1, and the newest segment has the index n: 1, 2,..., n\nwhere n is the number of acquired segments.\n\nAvailable Repeated Capabilities:\nMath: MA1, MA2, MA3, MA4, MA5\r\n\nRemote-control command(s):\nCALCulate:MATH<m>:HISTory:STOP"}, {"Level"=4, "Class Only"=FALSE, "Identifier"="RSRTX_ATTR_HISTORY_MATH_PLAY_ALL", "Descriptive Name"="History Math Play All", "Data Type"=3, "Command"="CALC:MATH{Math}:HIST:PALL", "Access"=2, "Range Table"="", "Read Callback"="", "Write Callback"="", "Supported Models"="RTM|RTA", "Instrument Options"="K15", "Flags"=0, "Help"="Enables the replay of all acquired segments.\n\nAvailable Repeated Capabilities:\nMath: MA1, MA2, MA3, MA4, MA5\r\n\nRemote-control command(s):\nCALCulate:MATH<m>:HISTory:PALL"}, {"Level"=4, "Class Only"=FALSE, "Identifier"="RSRTX_ATTR_HISTORY_MATH_SPEED", "Descriptive Name"="History Math Speed", "Data Type"=0, "Command"="CALC:MATH{Math}:HIST:PLAY:SPE", "Access"=2, "Range Table"="rsrtx_rngHistorySpeed", "Read Callback"="", "Write Callback"="", "Supported Models"="RTM|RTA", "Instrument Options"="K15", "Flags"=0, "Help"="Sets the speed of the history replay.\n\nAvailable Repeated Capabilities:\nMath: MA1, MA2, MA3, MA4, MA5\r\n\nRemote-control command(s):\nCALCulate:MATH<m>:HISTory:PLAYer:SPEed"}, {"Level"=4, "Class Only"=FALSE, "Identifier"="RSRTX_ATTR_HISTORY_MATH_REPEAT", "Descriptive Name"="History Math Repeat", "Data Type"=3, "Command"="CALC:MATH{Math}:HIST:REPL", "Access"=2, "Range Table"="", "Read Callback"="", "Write Callback"="", "Supported Models"="RTM|RTA", "Instrument Options"="K15", "Flags"=0, "Help"="If set to true, the replay of the selected history segments repeats automatically.\n\nAvailable Repeated Capabilities:\nMath: MA1, MA2, MA3, MA4, MA5\r\n\nRemote-control command(s):\nCALCulate:MATH<m>:HISTory:REPLay"}, {"Level"=4, "Class Only"=FALSE, "Identifier"="RSRTX_ATTR_HISTORY_MATH_ACQUISITON_RELATIVE_TIME", "Descriptive Name"="History Math Acquisiton Relative Time", "Data Type"=1, "Command"="CALC:MATH{Math}:HIST:TSR?", "Access"=0, "Range Table"="", "Read Callback"="", "Write Callback"="", "Supported Models"="RTM|RTA", "Instrument Options"="K15", "Flags"=0, "Help"="Returns the time difference of the selected segment to the newest segment.\n\nAvailable Repeated Capabilities:\nMath: MA1, MA2, MA3, MA4, MA5\r\n\nRemote-control command(s):\nCALCulate:MATH<m>:HISTory:TSRelative?"}, {"Level"=4, "Class Only"=FALSE, "Identifier"="RSRTX_ATTR_HISTORY_MATH_ALL_DATES", "Descriptive Name"="History Math All Dates", "Data Type"=2, "Command"="CALC:MATH{Math}:HIST:TSD:ALL?", "Access"=0, "Range Table"="", "Read Callback"="", "Write Callback"="", "Supported Models"="RTM|RTA", "Instrument Options"="", "Flags"=0, "Help"="Returns the dates of all history segments.\n\nAvailable Repeated Capabilities:\nMath: MA1, MA2, MA3, MA4, MA5\r\n\nRemote-control command(s):\nCALCulate:MATH<m>:HISTory:TSDate:ALL?"}, {"Level"=4, "Class Only"=FALSE, "Identifier"="RSRTX_ATTR_HISTORY_MATH_ALL_TIME_DIFFERENCES", "Descriptive Name"="History Math All Time Differences", "Data Type"=2, "Command"="CALC:MATH{Math}:HIST:TSR:ALL?", "Access"=0, "Range Table"="", "Read Callback"="", "Write Callback"="", "Supported Models"="RTM|RTA", "Instrument Options"="", "Flags"=0, "Help"="Returns the time differences to the newest acquisition of all history segments.\n\nAvailable Repeated Capabilities:\nMath: MA1, MA2, MA3, MA4, MA5\r\n\nRemote-control command(s):\nCALCulate:MATH<m>:HISTory:TSRelative:ALL?"}, {"Level"=4, "Class Only"=FALSE, "Identifier"="RSRTX_ATTR_HISTORY_MATH_ALL_DAYTIMES", "Descriptive Name"="History Math All Daytimes", "Data Type"=2, "Command"="CALC:MATH{Math}:HIST:TSAB:ALL?", "Access"=0, "Range Table"="", "Read Callback"="", "Write Callback"="", "Supported Models"="RTM|RTA", "Instrument Options"="", "Flags"=0, "Help"="Returns the absolute daytimes of all history segments.\n\nAvailable Repeated Capabilities:\nMath: MA1, MA2, MA3, MA4, MA5\r\n\nRemote-control command(s):\nCALCulate:MATH<m>:HISTory:TSABsolute:ALL?"}, {"Level"=4, "Class Only"=FALSE, "Identifier"="RSRTX_ATTR_HISTORY_MATH_PLAYER_CONTROL_ENABLE", "Descriptive Name"="History Math Player Control Enable", "Data Type"=3, "Command"="CALC:MATH{Math}:HIST:CONT", "Access"=2, "Range Table"="", "Read Callback"="", "Write Callback"="", "Supported Models"="", "Instrument Options"="K15", "Flags"=0, "Help"="Displays or hides the history player on the screen.\n\nAvailable Repeated Capabilities:\nMath: MA1, MA2, MA3, MA4, MA5\r\n\nRemote-control command(s):\nCALCulate:MATH<m>:HISTory:CONTrol[:ENABle]"}, {"Level"=4, "Class Only"=FALSE, "Identifier"="RSRTX_ATTR_HISTORY_MATH_TIME_TABLE_ENABLE", "Descriptive Name"="History Math Time Table Enable", "Data Type"=3, "Command"="CALC:MATH{Math}:HIST:TTAB", "Access"=2, "Range 
